vi "ROI to Target.vi"(11 "ROI":T1) -> (0 "E_y":dbl, 1 "E_x":dbl, 3 "Target Coordinates":dbl[](array[numeric]))   [LabVIEW 2018]
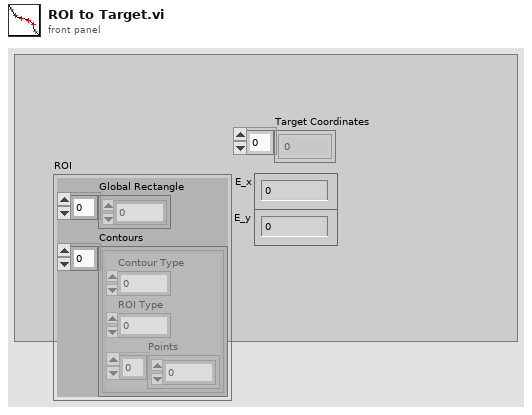
[diagram p1: front panel]
types:
  T1 = cluster{"Global Rectangle":i32[], "Contours":cluster{"Contour Type":u32, "ROI Type":u32, "Points":i32[]}[]}
  T2 = cluster{"Contour Type":u32, "ROI Type":u32, "Points":i32[]}[]
  T3 = cluster{"Contour Type":u32, "ROI Type":u32, "Points":i32[]}
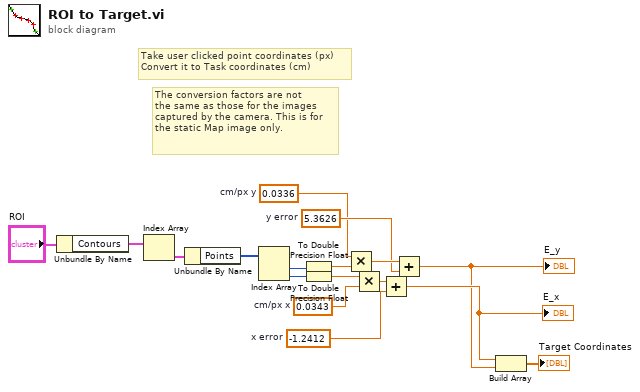
[diagram p0: block diagram]
diagram:
  w7 = 0.0336  # cm/px y
  w8 = -1.2412  # x error
  w12 = 0.0343  # cm/px x
  w9 = 5.3626  # y error
  # "The conversion factors are not \nthe same as those for the images\ncaptured by the camera. This is for\nthe static Map image only."
  # "Take user clicked point coordinates (px)\nConvert it to Task coordinates (cm)"
  n1 = Unbundle By Name("ROI") -> ("Contours"=w15:T2)
  n2 = Index Array(array=w15) -> (element=w6:T3)  [unwired: 1 in]
  n3 = Unbundle By Name(w6) -> ("Points"=w5:i32[])
  n4 = Index Array(array=w5) -> (element #1=w4:i32, element #2=w3:i32)  [unwired: 2 in]
  n5 = To Double Precision Float(number=w4) -> (double precision float=w14:dbl)
  n6 = To Double Precision Float(number=w3) -> (double precision float=w13:dbl)
  n7 = Multiply(x=w7, y=w14) -> (x*y=w11:dbl)
  n8 = Multiply(x=w13, y=w12) -> (x*y=w10:dbl)
  n9 = Add(x=w10, y=w8) -> (x+y=w2:dbl)
  "E_x" <- w2
  n10 = Add(x=w11, y=w9) -> (x+y=w1:dbl)
  "E_y" <- w1
  n11 = Build Array(w2, w1) -> (→"Target Coordinates":dbl[])
